vi "myK705C.vi"(0 "run?":bool, 1 "set up\nscanner?":bool, 2 "channels":bool[](array[boolean])=[FALSE, FALSE, FALSE, FALSE, FALSE, FALSE, FALSE, FALSE, FALSE, FALSE, FALSE, FALSE, FALSE, FALSE, FALSE, FALSE, FALSE, FALSE, FALSE, FALSE], 3 "scan mode \n (step:0)":i16(slide) scale=0.0..2.0 scale format="%.2f", 4 "interval(sec)":ext=0.01 format="%.3f", 5 "last channel":ext=1.0, 6 "first channel":ext=1.0, 7 "measurement poles\n  (1-pole 20ch:0)":i16(slide) scale=0.0..2.0) -> ()   [LabVIEW 2015]
doc: "Keithley 705 Scanner\n\nUse: Allows opening a selected channel, closing the channel, scanning between a selected first and last channel, selecting scan rate and mode, and selecting 1-, 2-, or 4-pole measurement modes.\n\nDefaults: \n Measurement Poles = 1-Pole, 20 channels/card First Channel = 1\n Last channel = 1 Interval(sec) = 10mS Scan Mode = Step Channels = All channels open Trigger Mode = Internal Set Up Scanner? = No\n Run? = No\n\nAssumptions: GPIB address = 17; the bus is properly connected.\n\nCapabilities not implemented: settling time of each channel; time; date; alarm time; saving/recalling of a relay set up; SRQ.\nThese capabilities can all be implemented by adding a numeric or slide control and adding the proper command code to the command string. The codes are located on pp. 3-9 to 3-11.\n\nInteractively:\n Measurement Poles - Select a measurement-poles mode. In 2-pole operation, each channel consists of a HI and a LO line. Since there are twenty different lines on a card, 2-pole operation has a maximum of ten channels per card. In 1-pole operation, the HI and LO lines are used independently; each line is one channel. Therefore, the maximum number of channels in the 1-pole mode is twenty.\nIn 4-pole operation, each channel uses four lines, two HI and two LO lines. Thus, it requires two cards to make ten channels.\n\n Card Possible measurement-pole modes\n 7056 General Purpole Scanner 1-pole and 2-pole\n 7057 Thermocouple Scanner 2-pole\n 7058 Low Current Scanner Plug-In Card 1-pole\n\n First Channel - Select a channel from 1 to 20 to be the starting channel of a scan.\n Last Channel - Select a channel from 1 to 20 to be the ending channel in a scan. Keep in mind that the last channel can never be less than the first channel.\n Interval(sec) - Enter a time from 5mS to 999.999S. This is the time each channel is closed when using the single, continuous, or step scanning modes.\n Scan Mode - Select a scan mode.\n Channels - Select and close the desired channels.\n Trigger Mode - Select trigger mode. External trigger allows manual triggering from the front panel of the 705 via the \"START/STOP\" button or signal triggering from the rear panel via the BNC connection.\n Set Up Scanner? - Select \"Yes\" when the user wants to change the present set up parameters of the scanner. This control is implemented independently of the \"Run?\" control so that the user can use the step scan mode without resetting the scanner parameters everytime the VI is run.\n Run? - Select \"Start\" to begin a scan from the present channel when using continuous or single scan mode or to step through the next channel when using the step scan mode. Select \"Stop\" to terminate in the middle of a scan.\n\nProgrammatically: There are 8 inputs. Trigger mode is the only control that cannot be programmed. All other controls can be programmed as described below.\n\nMeasurement Poles: 0 = 1-Pole, 20 ch/card 1 = 2-Pole, 10 ch/card 2 = 4-Pole, 10 ch/card\nFirst Channel: Numeric (range 1.. 20)\nLast Channel: Numeric (range 1.. 20)\nInterval(sec): Numeric (range 5mS to 999.999S)\nScan Mode: 0 = Step Scan 1 = Single scan 2 = Cont. scan\nChannels: Bit vector (Channel 1 is at bit 1. Ignore bit 0. Keithley 705 does not have a channel 0.)\nSet up scanner?: Binary\nRun?: Binary"
panel:
  in  "trigger\nmode":bool
  # "KEITHLEY 705 SCANNER"
  # "yes\n\nno"
  # "close\nopen"
  # "start\n\nstop"
  # "ext\nint"
  # "© Copyright 1993 National Instruments Corporation.  All Rights Reserved."
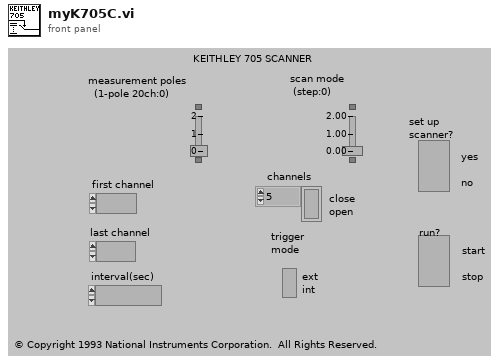
[diagram p1: front panel]
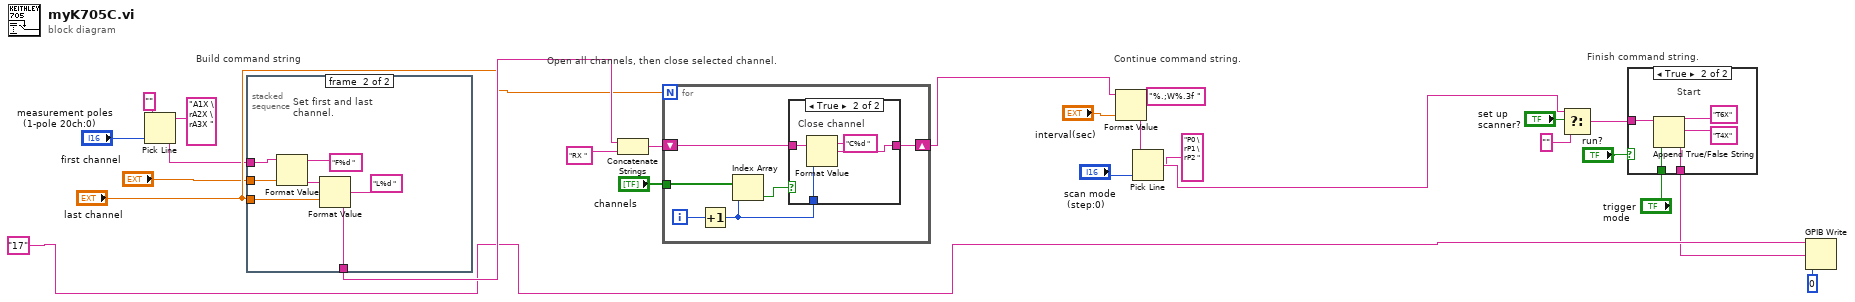
[diagram p0: block diagram]
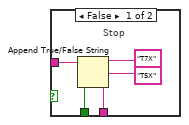
[diagram p2: hidden frame]
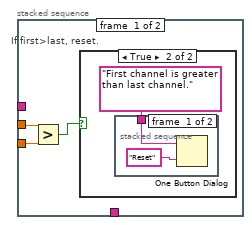
[diagram p4: hidden frame]
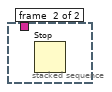
[diagram p6: hidden frame]
diagram:
  # "Finish command string."
  # "Continue command string."
  # "Open all channels, then close selected channel."
  # "Build command string"
  n1 = Pick Line(string ("")="", multi-line string="A1X \rA2X \rA3X ", line index="measurement poles\n  (1-pole 20ch:0)") -> (output string=w18:string)
  n2 = stacked-sequence {
    tunnel: w18 -> [_ w32]
    tunnel: "first channel" -> [w26 w34]
    tunnel: "last channel" -> [w27 w35]
    tunnel: [_ w38] -> w25
    frame #0 {
      # "If first>last, reset."
      n3 = Greater?(x=w26, y=w27) -> (0:w28:bool)
      n4 = case shown="True" w28 {
        frame False {
        }
        frame True {
          n5 = stacked-sequence {
            tunnel: "First channel is greater than last channel." -> [w30 _]
            frame #0 {
              n6 = One Button Dialog(message=w30, button name ("OK")="Reset") -> ()  [unwired: 1 out]
            }
            frame #1 {
              n7 = Stop() -> ()  [unwired: 1 in]
            }
          }
        }
      }
    }
    frame #1 {
      # "Set first and last\nchannel."
      n8 = Format Value(string ("")=w32, format string="F%d ", value (0)=w34) -> (output string=w36:string)
      n9 = Format Value(string ("")=w36, format string="L%d ", value (0)=w35) -> (output string=w38:string)
    }
  }
  n10 = Concatenate Strings(w25, "RX ") -> (w15:string)
  n11 = for {
    N: "last channel" -> [_]
    shift-right: [w44] -> w23
    shift-left: w15 -> [w43]
    tunnel: "channels" -> [w40]
    i -> [w39]
    n12 = Increment(x=w39) -> (x+1=w42:i32)
    n13 = Index Array(array=w40, index=w42) -> (element=w41:bool)
    n14 = case shown="True" w41 {
      tunnel: w43 -> [w45 w46]
      tunnel: w42 -> [_ w47]
      tunnel: [w45 w49] -> w44
      frame False {
        # "Leave channel\n    open"
      }
      frame True {
        # "Close channel"
        n15 = Format Value(string ("")=w46, format string="C%d ", value (0)=w47) -> (output string=w49:string)
      }
    }
  }
  n16 = Format Value(string ("")=w23, format string="%.;W%.3f ", value (0)="interval(sec)") -> (output string=w10:string)
  n17 = Pick Line(string ("")=w10, multi-line string="P0 \rP1 \rP2 ", line index="scan mode \n (step:0)") -> (output string=w21:string)
  n18 = Select(t=w21, s="set up\nscanner?", f="") -> (s? t:f=w5:string)
  n19 = case shown="True" "run?" {
    tunnel: w5 -> [w50 w55]
    tunnel: "trigger\nmode" -> [w51 w59]
    tunnel: [w54 w58] -> w7
    frame False {
      # "Stop"
      n20 = Append True/False String(1:w51, 2:"T5X", 3:"T7X", 4:w50) -> (0:w54:string)
    }
    frame True {
      # "Start"
      n21 = Append True/False String(1:w59, 2:"T4X", 3:"T6X", 4:w55) -> (0:w58:string)
    }
  }
  n22 = GPIB Write(0:"17", 1:w7, 2:0) -> ()  [unwired: 2 in, 2 out]
